vi "SiggenSetAmpl.vi"(2 "error in (no error)":errorcluster, 3 "Amplitude request (dBm)":dbl=-80.0 min=-120.0 max=20.0 step=0.02 format="%#_9g") -> (0 "error out":errorcluster, 1 "Ampl returned (dBm)":dbl format="%#_8f")   [LabVIEW 2009]
doc: "Sets the amplitude on the siggen.\nReads back the amplitude as set by the siggen."
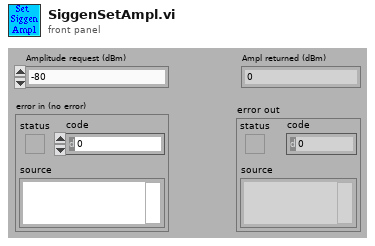
[diagram p1: front panel]
types:
  T1 = enum16{"N1911A", "Siggen", "34980a", "E4418B", "Rvp8"}
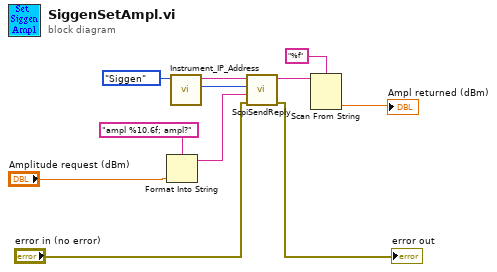
[diagram p0: block diagram]
diagram:
  n1 = Format Into String(format string="ampl %10.6f; ampl?", "Amplitude request (dBm)") -> (resulting string=w9:string)  [unwired: 2 in, 1 out]
  n2 = call "Instrument_IP_Address.vi"("Instrument"=T1."Siggen") -> ("Port"=w1:u16, "IP Address"=w2:string)  [unwired: 9 in]
  n3 = call "ScpiSendReply.vi"("error in (no error)"="error in (no error)", "Command"=w9, "TCP port"=w1, "IP Address"=w2) -> ("Error out"=→"error out":errorcluster, "Reply"=w6:string)  [unwired: 5 in]
  n4 = Scan From String(format string="%f", input string=w6) -> (output 1=→"Ampl returned (dBm)":dbl)  [unwired: 3 in, 3 out]
